vi "Element Type.vi"(11 "SystemConfigStatusIndicator in":refnum<class "SystemConfigStatusIndicator.lvclass">) -> (2 "Element Type":string)   [LabVIEW 2020, in "VolatusGUIElements.lvlib" / "SystemConfigStatusIndicator.lvclass"]
uses:
  SystemConfigStatusIndicator.lvclass
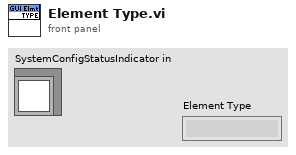
[diagram p1: front panel]
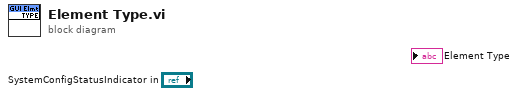
[diagram p0: block diagram]
diagram:
